vi "FilePacketRoutedMessage_Parse.vi"(8 "error in (no error)":errorcluster, 11 "Message":T5) -> (0 "error out":errorcluster, 1 "FilePacket":T4, 2 "Header":T2, 3 "FilePacketRoutedMessage":T1)   [LabVIEW 2017]
uses:
  <vilib>/addons/InsightCM/MessageBus/Base/controls/Message.ctl
  <vilib>/addons/InsightCM/MessageBus/Base/controls/MessageHeader.ctl
  <vilib>/addons/InsightCM/MessageBus/Base/controls/KeyValuePair.ctl
  <vilib>/addons/InsightCM/MessageBus/Base/controls/FilePacket.ctl
  <vilib>/addons/InsightCM/MessageBus/MessageLibrary/FileIngestion/controls/FilePacketRoutedMessage.ctl
  <vilib>/addons/InsightCM/Utilities/PropertyHelpers/PropertyHelpers.lvlib
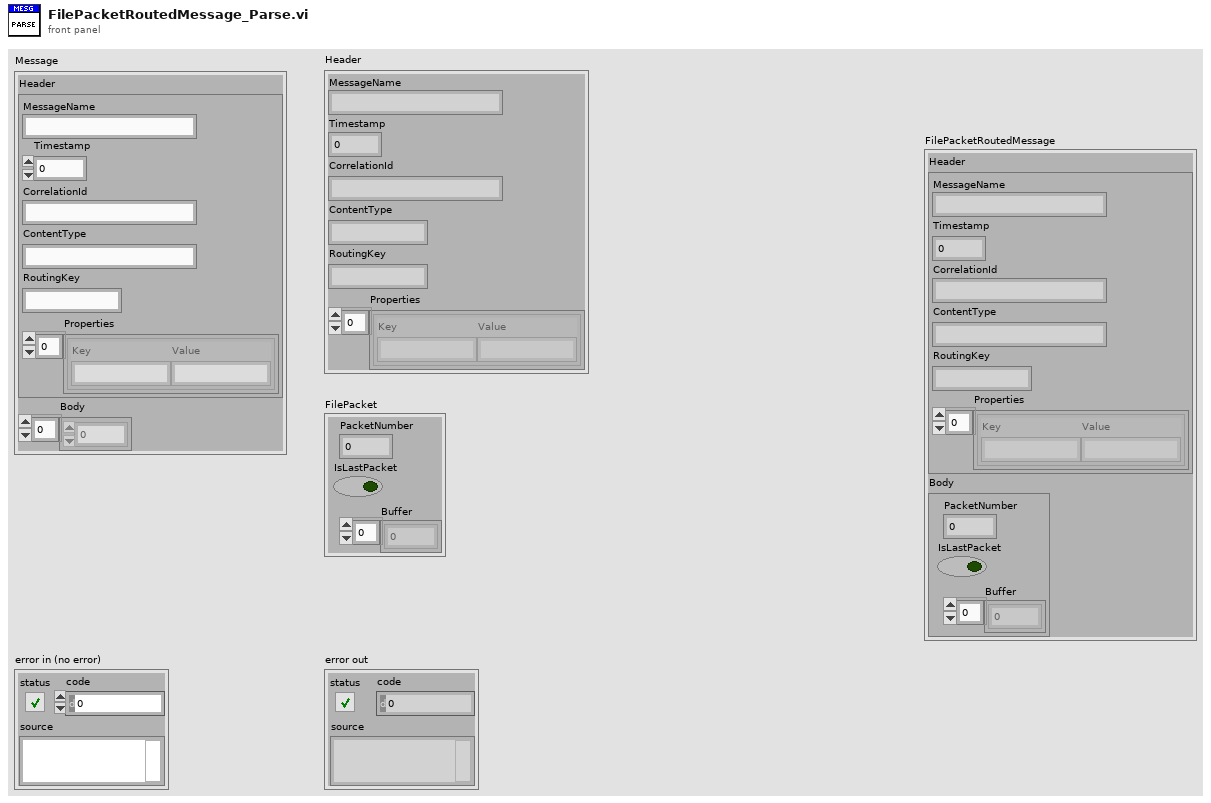
[diagram p1: front panel]
types:
  T1 = typedef "FilePacketRoutedMessage.ctl" = cluster{"Header":T2, "Body":T4}
  T2 = typedef "MessageHeader.ctl" = cluster{"MessageName":string, "Timestamp":i64, "CorrelationId":string, "ContentType":string, "RoutingKey":string, "Properties":T3[]}
  T3 = typedef "KeyValuePair.ctl" = cluster{"Key":string, "Value":string}
  T4 = typedef "FilePacket.ctl" = cluster{"PacketNumber":i32, "IsLastPacket":bool, "Buffer":u8[]}
  T5 = typedef "Message.ctl" = cluster{"Header":T2, "Body":u8[]}
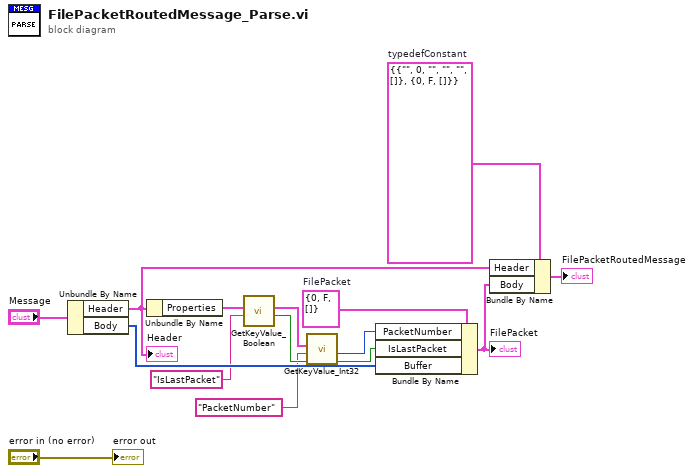
[diagram p0: block diagram]
diagram:
  w10 = T1 {"Header"={"MessageName"="", "Timestamp"=0, "CorrelationId"="", "ContentType"="", "RoutingKey"="", "Properties"=[]}, "Body"={"PacketNumber"=0, "IsLastPacket"=FALSE, "Buffer"=[]}}  # typedefConstant
  w11 = T4 {"PacketNumber"=0, "IsLastPacket"=FALSE, "Buffer"=[]}  # FilePacket
  n1 = Unbundle By Name("Message") -> ("Header"=w13:T2, "Body"=w7:u8[])
  "Header" <- w13
  n2 = Unbundle By Name(w13) -> ("Properties"=w6:T3[])
  n3 = call <vilib>:"GetKeyValue_Boolean.vi"("key"="IsLastPacket" ("Key"), "key value pairs"=w6) -> ("value"=w4:bool, "key value pairs out"=w3:T3[])  [unwired: 7 in, 1 out]
  n4 = call <vilib>:"GetKeyValue_Int32.vi"("key"="PacketNumber" ("Key"), "key value pairs"=w3) -> ("value"=w2:i32)  [unwired: 7 in, 2 out]
  n5 = Bundle By Name(cluster=w11, "PacketNumber"=w2, "IsLastPacket"=w4, "Buffer"=w7) -> (w9:T4)
  "FilePacket" <- w9
  n6 = Bundle By Name(cluster=w10, "Header"=w13, "Body"=w9) -> (→"FilePacketRoutedMessage":T1)
  "error out" <- "error in (no error)"
